vi "KE2182 Voltage.vi"() -> ()   [LabVIEW 2018]
panel:
  out "KE2182 Voltage (V)":dbl
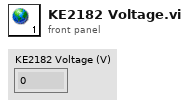
[diagram p1: front panel]
diagram:
